vi "Init.vi"(8 "error in (no error)":errorcluster, 9 "Config File Path":path=path "", 10 "Name":string, 11 "Process In":refnum<class "Process.lvclass">) -> (0 "error out":errorcluster, 3 "Process Out":refnum<class "Process.lvclass">)   [LabVIEW 2020, in "Process.lvclass"]
doc: "Initializes the process and creates necessary references. Anything initialized here is released in the Clear.vi method."
uses:
  Process.lvclass
  Protected/Messaging/Message Cluster.ctl
  Process.lvclass/Process.ctl
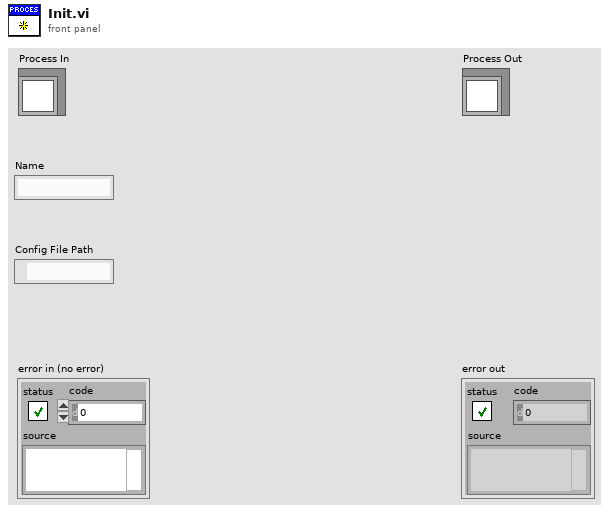
[diagram p1: front panel]
types:
  T1 = typedef "Process.lvclass/Message Cluster.ctl" = cluster{"Message":string, "Message Data":variant}
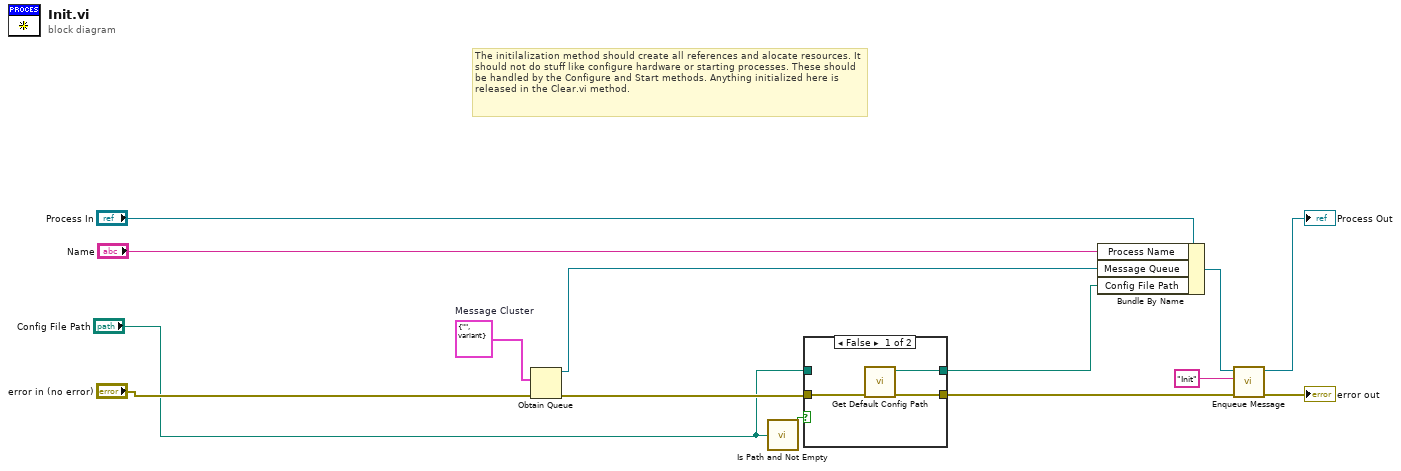
[diagram p0: block diagram]
diagram:
  w5 = T1 {"Message"="", "Message Data"=variant}  # Message Cluster
  # "The initilalization method should create all references and alocate resources. It should not do stuff like configure hardware or starting processes. These should be handled by the Configure and Start methods. Anything initialized here is released in the Clear.vi method."
  n1 = Obtain Queue(element data type=w5, error in (no error)="error in (no error)") -> (queue out=w13:refnum<queue>, error out=w12:errorcluster)  [unwired: 3 in, 1 out]
  n2 = call <vilib>:"Is Path and Not Empty.vi"("path"="Config File Path") -> ("Is Path and Not Empty?"=w3:bool)  [unwired: 4 in]
  n3 = case shown="False" w3 {
    tunnel: w12 -> [w17 w18]
    tunnel: [w16 w18] -> w4
    tunnel: [w15 w19] -> w2
    tunnel: "Config File Path" -> [_ w19]
    frame False {
      n4 = call "Get Default Config Path.vi"("error in (no error)"=w17) -> ("error out"=w16:errorcluster, "appended path"=w15:path)  [unwired: 9 in]
    }
    frame True {
    }
  }
  n5 = Bundle By Name(cluster="Process In", "Process Name"="Name", "Message Queue"=w13, "Config File Path"=w2) -> (w14:refnum<class "Process.lvclass">)
  n6 = call "Enqueue Message.vi"("error in (no error)"=w4, "Message"="Init", "Process In"=w14) -> ("error out"=→"error out":errorcluster, "Process Out"=→"Process Out":refnum<class "Process.lvclass">)  [unwired: 7 in]
